vi "Stop Core.vi"(10 "final error code":i32, 11 "[V]System Tree View in":refnum<class "[V]System Tree View.lvclass">) -> (3 "[V]System Tree View out":refnum<class "[V]System Tree View.lvclass">)   [LabVIEW 2020, in "[V]System Tree View.lvlib" / "[V]System Tree View.lvclass"]
doc: "(<B>Filename</B>: Actor Framework.lvlib:Actor.lvclass:Stop Core.vi)\n\nDefines what the actor does before it stops. Use the <B>final error code</B> input to determine whether the actor shut down in response to an error.\n\nBy default, this method passes the Stop message along to all auto-stop nested actors. A descendant class may override this method to define additional behavior, such as shutting down any processes the actor initiated in its override of the Actor Core method."
uses:
  [V]System Tree View.lvclass
  MVVM Framework/MVVM Abstruct View/MVVM Abstruct View/MVVM Abstruct View.lvclass
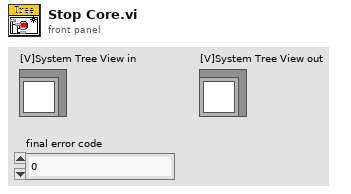
[diagram p1: front panel]
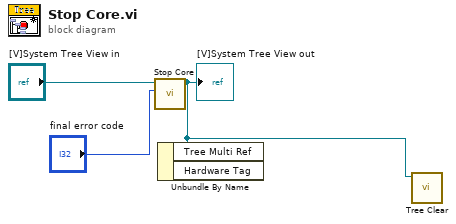
[diagram p0: block diagram]
diagram:
  n1 = call-parent "Stop Core.vi"("final error code"="final error code", "Abstruct View in"="[V]System Tree View in") -> ("Abstruct View out"=w1:refnum<class "[V]System Tree View.lvclass">)  [unwired: 9 in]
  "[V]System Tree View out" <- w1
  n2 = Unbundle By Name(w1) -> ()  [unwired: 2 out]
  n3 = call "Tree Clear.vi"("[V]System Tree View in"=w1) -> ()  [unwired: 9 in, 2 out]
